vi "Enqueue Multiple.vi"(8 "error in (no error)":errorcluster, 10 "Array":string[](array[string]), 11 "Queue in":refnum<queue>) -> (0 "error out":errorcluster)   [LabVIEW 2016, in "Intake.lvlib"]
uses:
  Intake.lvlib
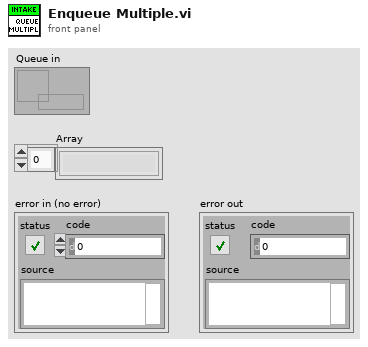
[diagram p1: front panel]
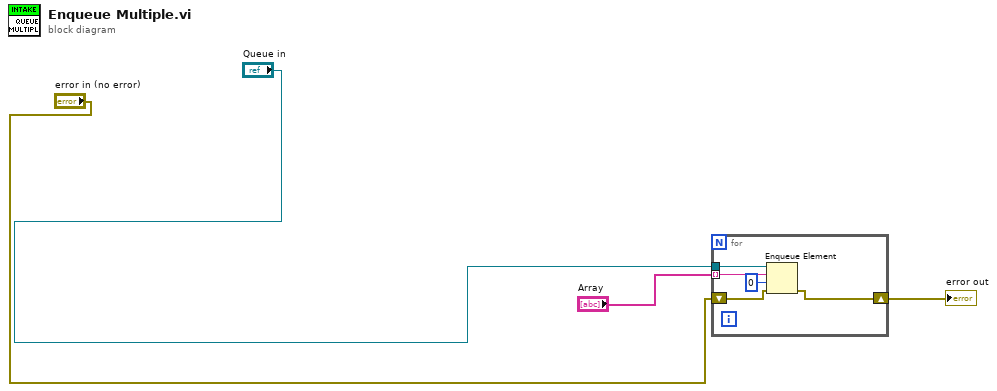
[diagram p0: block diagram]
diagram:
  n1 = for {
    tunnel: "Queue in" -> [w9]
    tunnel: "Array" -> [w8] mode=indexing
    shift-right: [w5] -> w4
    shift-left: "error in (no error)" -> [w6]
    n2 = Enqueue Element(queue=w9, element=w8, timeout in ms (-1)=0, error in (no error)=w6) -> (error out=w5:errorcluster)  [unwired: 2 out]
  }
  "error out" <- w4
